vi "Host.vi"() -> ()   [LabVIEW 2018]
uses:
  Speciality IO/Types/Static.Generate.Digital.Settings.ctl
  Speciality IO/Types/Static.Measure.Digital.Measurement.ctl
  Speciality IO/Types/PWM.Measure.Digital.Result.ctl
  Speciality IO/Types/PWM.Generate.Digital.Convert.Settings.ctl
  cbca53a3-fff1-474c-b426-55f8608b9b00.vi
  cRIO RT/FPGA Bitfile Register Operations/Scalar IO Operations/SubVIs/Check Cluster Configuration Store.vi
  cRIO RT/FPGA Bitfile Register Operations/Scalar IO Operations/SubVIs/DBL to FXP Raw.vi
  cRIO RT/FPGA Bitfile Register Operations/Scalar IO Operations/SubVIs/Convert Bool Array to Cluster BLOB.vi
  <userlib>/_OpenG.lib/lvdata/lvdata.llb/Variant to Header Info__ogtk.vi
  <userlib>/_OpenG.lib/lvdata/lvdata.llb/Split Cluster TD__ogtk.vi
  <userlib>/_OpenG.lib/lvdata/lvdata.llb/Cluster to Array of VData__ogtk.vi
  <vilib>/Utility/Data Type/Get Type Information.vi
  <userlib>/_OpenG.lib/lvdata/lvdata.llb/Get Strings from Enum__ogtk.vi
  cRIO RT/FPGA Bitfile Register Operations/Scalar IO Operations/Error Handling/Error 6004.vi
  <vilib>/Utility/Data Type/Get Fixed-Point Information.vi
  cRIO RT/FPGA Bitfile Register Operations/Scalar IO Operations/FPGA Register IO.lvlib
  288c4aec-35d2-47aa-9a2b-ac8d79241408.vi
  66cdeb6e-13d4-4795-bea6-33fe6644b298.vi
  Speciality IO/Speciality FPGA IO.lvlib
panel:
  out "Array 2":u8[](array[numeric])
  out "bparray":u32[](array[numeric])
  out "Cluster Bool Data":bool[](array[boolean])
  out "Cluster array":bool[](array[boolean])
  out "bpacked array":bool[](array[boolean])
  out "Array":u8[](array[numeric])
  out "Cluster Byte Data":u8[](array[numeric])
  in  "Measurement":T1
  in  "Settings":T2={"ACTIVE EDGE"=TRUE, "OUTPUT"=FALSE}
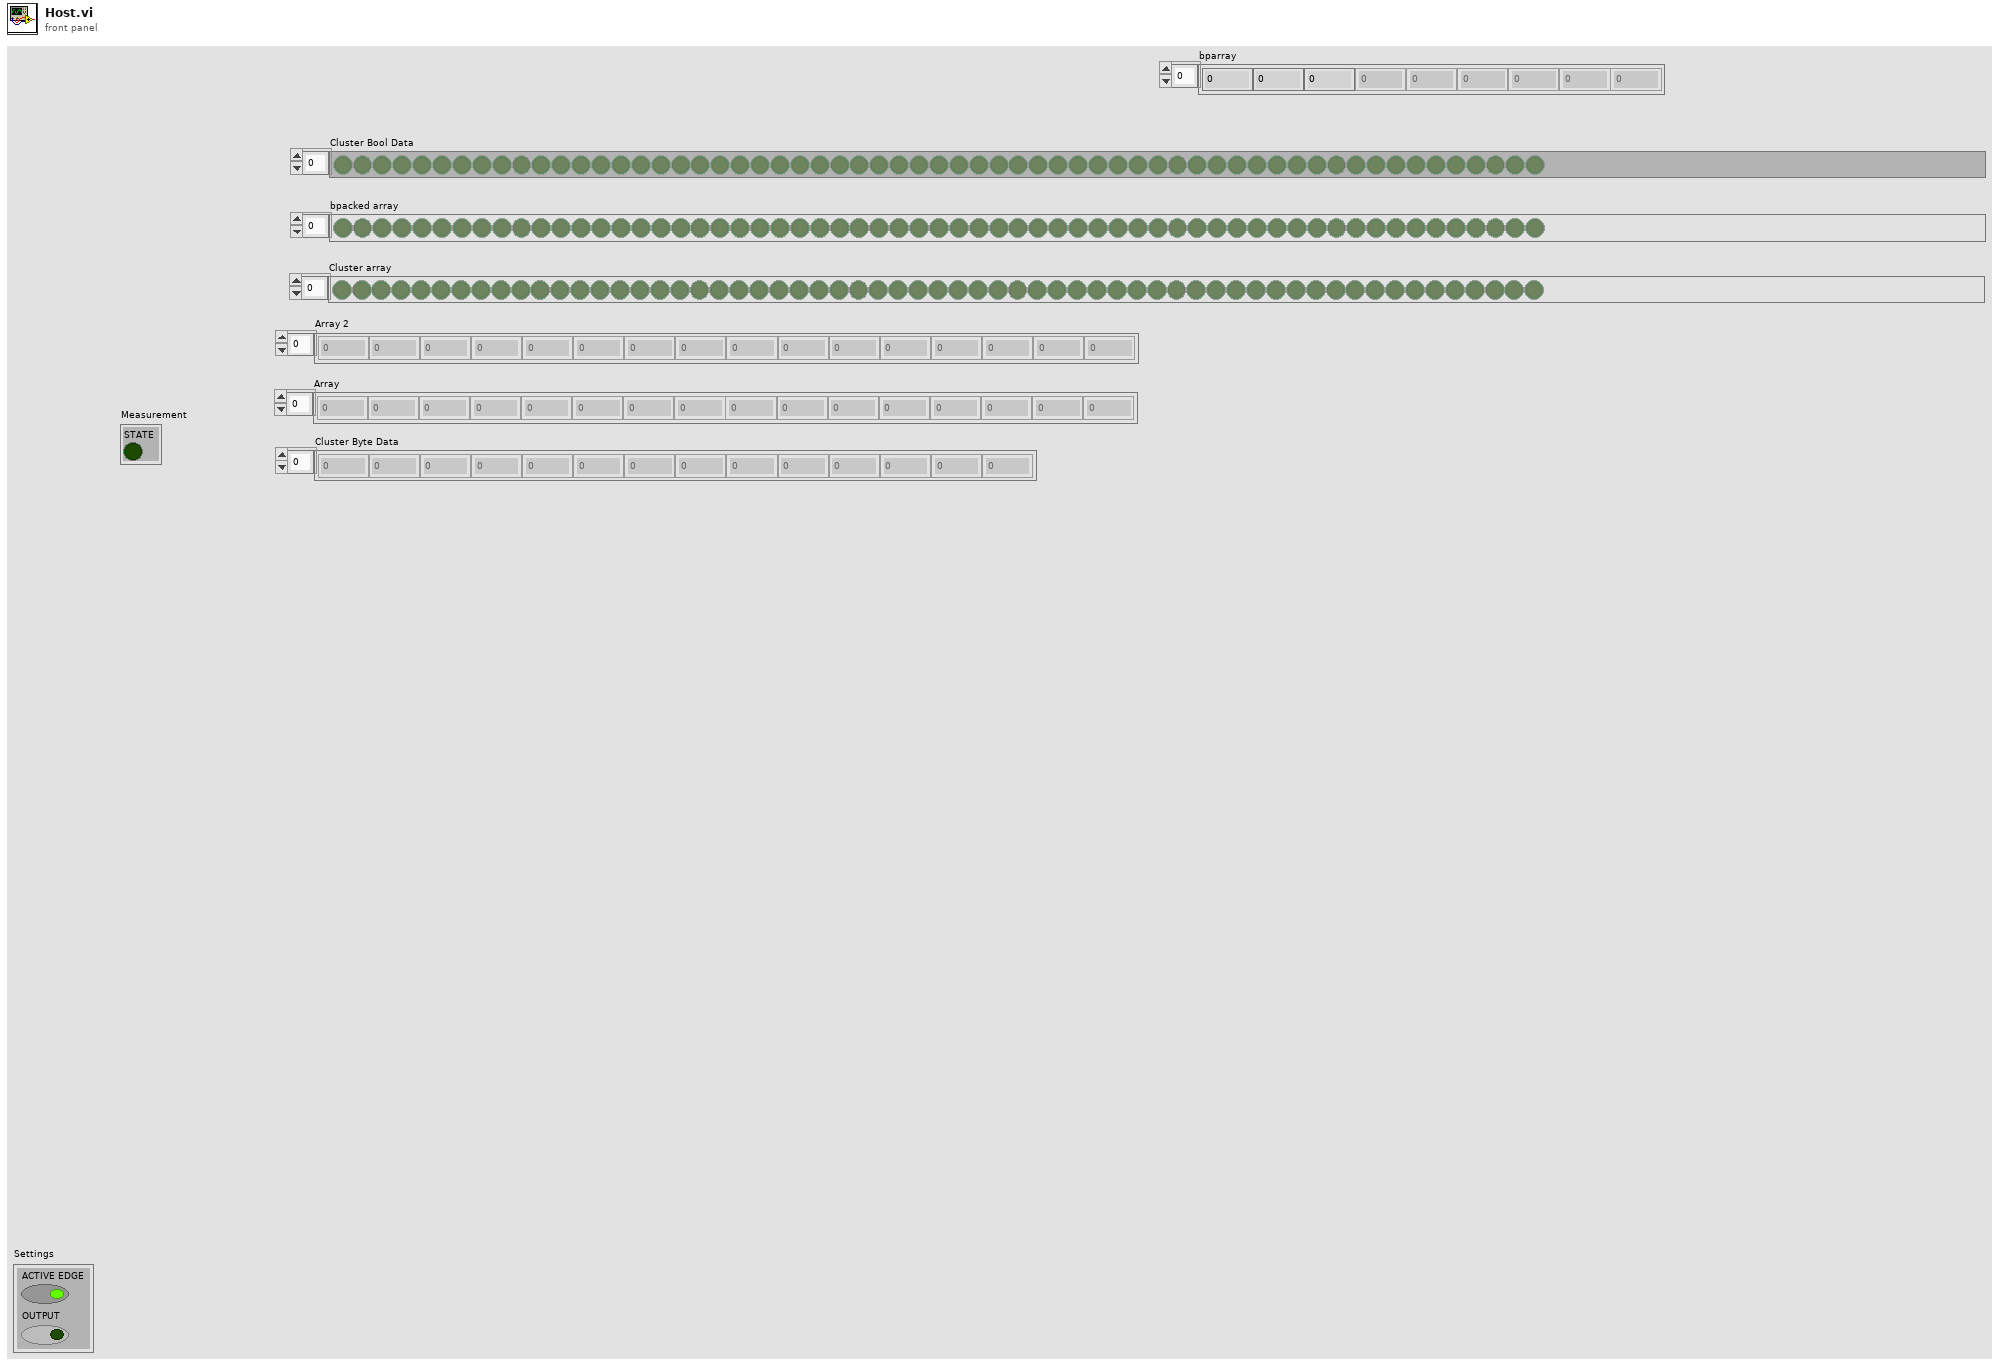
[diagram p1: front panel]
types:
  T1 = typedef "Speciality FPGA IO.lvlib/Static.Measure.Digital.Measurement.ctl" = cluster{"STATE":bool}
  T2 = typedef "Speciality FPGA IO.lvlib/Static.Generate.Digital.Settings.ctl" = cluster{"ACTIVE EDGE":bool, "OUTPUT":bool}
  T3 = typedef "Speciality FPGA IO.lvlib/PWM.Generate.Digital.Convert.Settings.ctl" = cluster{"ACTIVE EDGE":bool, "FREQ":sgl, "DC":sgl}
  T4 = cluster{"ACTIVE EDGE":bool, "FREQ":sgl, "DC":sgl, "ACTIVE EDGE 2":bool, "ACTIVE EDGE 3":bool}
  T5 = typedef "Speciality FPGA IO.lvlib/PWM.Measure.Digital.Result.ctl" = cluster{"FREQ":sgl, "PERIOD":sgl, "DC":sgl, "ACTIVE TIME":sgl}
  T6 = typedef "FPGA Register IO.lvlib/Cluster Configuration.ctl" = cluster{"Register Name":string, "Total Bits":i32, "Total Bytes":i32, "FPGA Start Indexes":i32[], "LV Start Indexes":i32[], "FPGA Data Sizes":i32[], "LV Data Sizes":i32[], "Type Descriptor":T7, "Element Type Descriptors":cluster{"Type Descriptor":T7}[], "Element Types":T8[], "Element Data Strings":string[], "Attributes":variant[], "Cluster VData Array":variant[], "Bool Array":bool[], "Byte Array":u8[]}
  T7 = typedef "Type Descriptor__ogtk.ctl" = i16[]
  T8 = typedef "NI_Data Type.lvlib/Data Type.ctl" = enum8{"Invalid Type", "Void", "I8", "I16", "I32", "I64", "U8", "U16", "U32", "U64", "Single Float", "Double Float", "Extended Float", "Single Complex", "Double Complex", "Extended Complex", "Enum U8", "Enum U16", "Enum U32", "Enum U64", "Single Float With Unit", "Double Float With Unit", "Extended Float With Unit", "Single Complex with Unit", "Double Complex with Unit", "Extended Complex with Unit", "Boolean", "String", "Path", "Picture", "Tag", "Array", "Cluster", "Variant", "LV Variant", "Waveform", "Timestamp", "Digital Waveform", "Digital Data", "ExpressData", "Refnum", "External Data", "VI", "Poly VI", "LabVIEW Class Instance", "Fixed Point"}
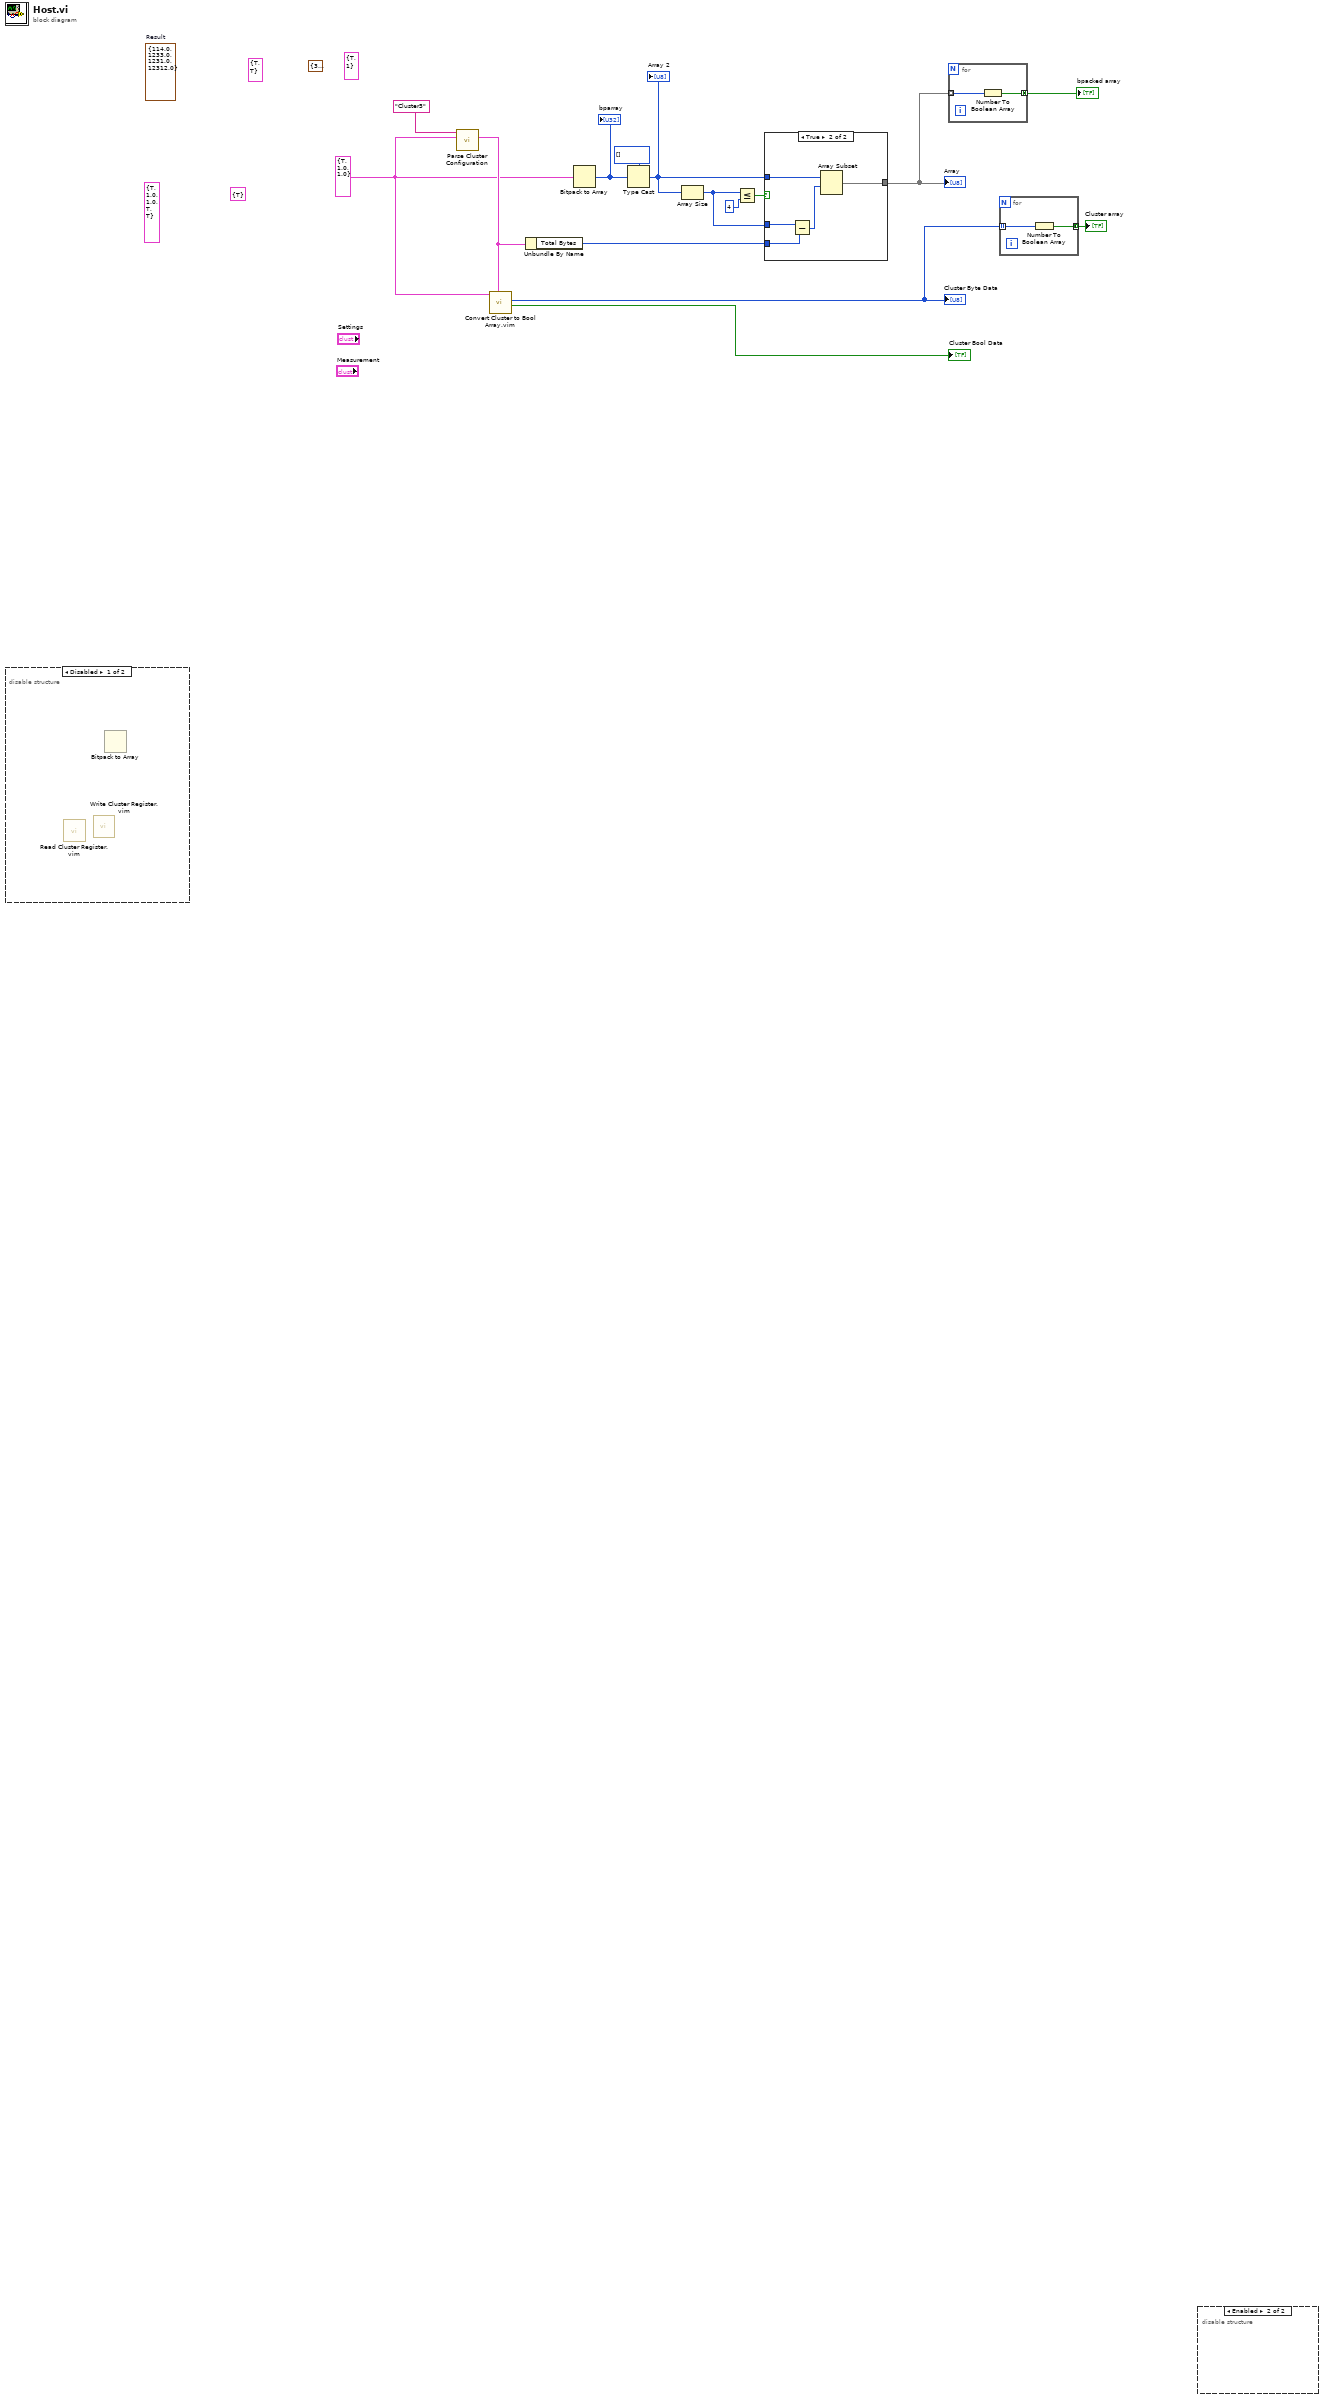
[diagram p0: block diagram]
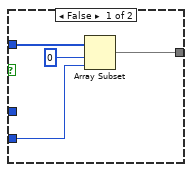
[diagram p2: hidden frame]
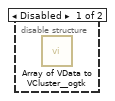
[diagram p4: hidden frame]
diagram:
  w1 = T3 {"ACTIVE EDGE"=TRUE, "FREQ"=1.0, "DC"=1.0} ("Digital Convert Settings out")
  (unwired) T1 {"STATE"=TRUE} ("Measurement")
  (unwired) T2 {"ACTIVE EDGE"=TRUE, "OUTPUT"=TRUE} ("Settings")
  (unwired) cluster{"ACTIVE EDGE":bool, "FREQ":i8} {"ACTIVE EDGE"=TRUE, "FREQ"=1}
  (unwired) cluster{"DC":i16} {"DC"=32767}
  (unwired) T4 {"ACTIVE EDGE"=TRUE, "FREQ"=1.0, "DC"=1.0, "ACTIVE EDGE 2"=TRUE, "ACTIVE EDGE 3"=TRUE} ("Digital Convert Settings out")
  (unwired) T5 {"FREQ"=114.0, "PERIOD"=1233.0, "DC"=1231.0, "ACTIVE TIME"=12312.0}  # Result
  n1 = disable-structure shown="Disabled" {
    frame Disabled {
      n2 = call "Read Cluster Register.vim"() -> ()  [unwired: 8 in, 4 out]
      n3 = call "Write Cluster Register.vim"() -> ()  [unwired: 10 in, 2 out]
      n4 = Bitpack to Array() -> ()  [unwired: 1 in, 1 out]
    }
    frame Enabled {
    }
  }
  n5 = call "Parse Cluster Configuration.vi"("Cluster in"=w1, "Register Name in"="Cluster3") -> ("Cluster Configuration"=w12:T6)  [unwired: 8 in, 1 out]
  n6 = call "Convert Cluster to Bool Array.vim"("Cluster Configuration"=w12, "Cluster in"=w1) -> ("Cluster Bool Data"=→"Cluster Bool Data":bool[], "Cluster Byte Data"=w5:u8[])  [unwired: 6 in, 2 out]
  "Cluster Byte Data" <- w5
  n7 = Unbundle By Name(w12) -> ("Total Bytes"=w14:i32)
  n8 = Bitpack to Array(1:w1) -> (0:w11:u32[])
  "bparray" <- w11
  n9 = Type Cast(type=u8[] [] ("Cluster Byte Data"), x=w11) -> (*(type *) &x=w2:u8[])
  "Array 2" <- w2
  n10 = Array Size(array=w2) -> (size(s)=w8:i32)
  n11 = Less Or Equal?(x=w8, y=4) -> (x <= y?=w9:bool)
  n12 = case shown="True" w9 {
    tunnel: w14 -> [w18 w23]
    tunnel: w2 -> [w19 w22]
    tunnel: w8 -> [_ w21]
    tunnel: [w16 w20] -> w7
    frame False {
      n13 = Array Subset(array=w19, index=0, length=w18) -> (w16:u8[])
    }
    frame True {
      n14 = Subtract(x=w21, y=w23) -> (x-y=w24:i32)
      n15 = Array Subset(array=w22, index=w24) -> (w20:u8[])  [unwired: 1 in]
    }
  }
  "Array" <- w7
  n16 = for {
    tunnel: w7 -> [w26] mode=indexing
    tunnel: [w25] -> w6 mode=concatenating
    n17 = Number To Boolean Array(number=w26) -> (Boolean array=w25:bool[])
  }
  "bpacked array" <- w6
  n18 = for {
    tunnel: w5 -> [w28] mode=indexing
    tunnel: [w27] -> w4 mode=concatenating
    n19 = Number To Boolean Array(number=w28) -> (Boolean array=w27:bool[])
  }
  "Cluster array" <- w4
  n20 = disable-structure shown="Enabled" {
    frame Disabled {
      n21 = call <userlib>:"Array of VData to VCluster__ogtk.vi"() -> ()  [unwired: 10 in, 2 out]
    }
    frame Enabled {
    }
  }
